vi "wait for plc bit.vi"(7 "inverse":bool, 8 "error in":errorcluster, 9 "tag":T2 {"DataSocket Reference"."OnStatusUpdated" format="%.0x"; "DataSocket Reference"."OnDataUpdated" format="%.0x"}, 11 "Abort Test":T1) -> (0 "error out":errorcluster, 3 "final values":bool)   [LabVIEW 2018]
uses:
  05.UserVI's/type defs/plc path and tag.ctl
  <vilib>/Platform/dataskt.llb/DataSocket Reference Type.ctl
  05.UserVI's/type defs/EOL Global Digital Input Control.ctl
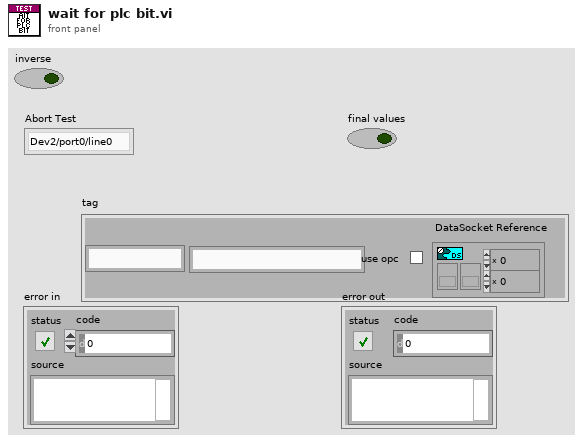
[diagram p1: front panel]
types:
  T1 = typedef "EOL Global Digital Input Control.ctl" = enum16{"Dev2/port0/line0", "Dev2/port0/line1", "Dev2/port0/line2", "Dev2/port0/line3", "Dev2/port0/line4", "Dev2/port0/line5", "Dev2/port0/line6", "Dev2/port0/line7", "Dev2/port1/line0", "Dev2/port1/line1", "Dev2/port1/line2", "Dev2/port1/line3", "Dev2/port1/line4", "Dev2/port1/line5", "Dev2/port1/line6", "Dev2/port1/line7", "Dev2/port2/line0", "Dev2/port2/line1", "Dev2/port2/line2", "Dev2/port2/line3", "Dev2/port2/line4", "Dev2/port2/line5", "Dev2/port2/line6", "Dev2/port2/line7", "Prerun Start Test", "Prerun Abort Test", "Audit Start Test", "Audit Abort Test", "Dev2/port3/line4", "Dev2/port3/line5", "Breakin Start Test", "Breakin Abort Test", "Not Implemented"}
  T2 = typedef "plc path and tag.ctl" = cluster{"Tag Name":string, "Network Path":string, "use opc":bool, "DataSocket Reference":T3}
  T3 = typedef "DataSocket Reference Type.ctl" = cluster{"CWDSLib._DCWDataSocket":refnum<k7>, "CWDSLib._DCWData":refnum<k7>, "OnDataUpdated":u32, "OnStatusUpdated":u32}
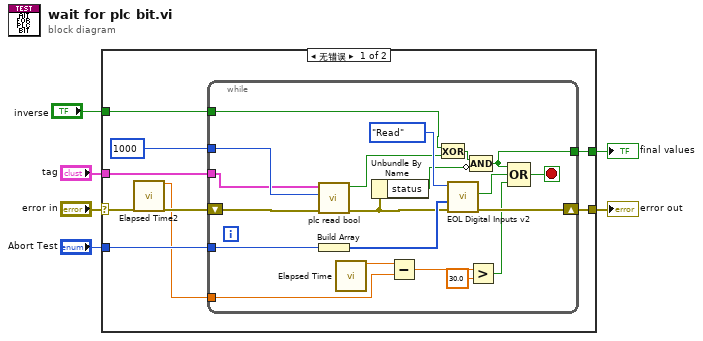
[diagram p0: block diagram]
diagram:
  n1 = case shown="无错误" "error in" {
    selector: "error in" -> [w9 w36]
    tunnel: "tag" -> [w15 _]
    tunnel: "Abort Test" -> [w14 _]
    tunnel: [w13 w36] -> w4
    tunnel: [w12 _] -> w3
    tunnel: "inverse" -> [w10 _]
    frame No Error {
      n2 = call "Elapsed Time2"("error in (no error)"=w9) -> ("Present (s)"=w7:dbl, "error out"=w8:errorcluster)  [unwired: 11 in, 6 out]
      n3 = while {
        tunnel: [w22] -> w12
        shift-right: [w34] -> w13
        shift-left: w8 -> [w29]
        tunnel: w14 -> [w33]
        tunnel: w15 -> [w27]
        tunnel: 1000 ("milliseconds to wait") -> [w28]
        tunnel: w10 -> [w30]
        tunnel: w7 -> [w18]
        stop <- w20 stop-if-true
        n4 = call "plc read bool.vi"("error in"=w29, "Timeout (ms)"=w28, "addr,tag"=w27) -> ("error out"=w25:errorcluster, "value"=w26:bool)  [unwired: 7 in]
        n5 = Build Array(w33) -> (w32:T1[])
        n6 = call "Elapsed Time"() -> ("Present (s)"=w19:dbl)  [unwired: 12 in, 7 out]
        n7 = Unbundle By Name(w25) -> ("status"=w24:bool)
        n8 = Subtract(x=w19, y=w18) -> (x-y=w17:dbl)
        n9 = Exclusive Or(1:w26, 2:w30) -> (0:w31:bool)
        n10 = call "EOL Digital Inputs v2.vi"("Sys Error In"=w25, "Digital Inputs Array"=w32, "Mode"=enum16{"Init", "Read", "Read All", "Close"}."Read") -> ("Sys Error Out"=w34:errorcluster, "Single Input"=w21:bool)  [unwired: 6 in, 1 out]
        n11 = Greater?(x=w17, y=30.0) -> (0:w16:bool)
        n12 = Compound Arithmetic op=AND(w31, invert w24) -> (w22:bool)
        n13 = Compound Arithmetic op=OR(w22, w21, w16) -> (w20:bool)
      }
    }
    frame Error {
    }
  }
  "error out" <- w4
  "final values" <- w3
